vi "Insert data.vi"(8 "error in":errorcluster, 9 "Seleccion":T2, 10 "variant":variant, 11 "url":string) -> (0 "error out":errorcluster)   [LabVIEW 2018]
uses:
  Seleccion.ctl
  Valores Zapato.ctl
  Valores venta almacen.ctl
  Modelo color.ctl
  <vilib>/httpClient/POSTBuffer.vi
  <vilib>/httpClient/LabVIEWHTTPClient.lvlib
panel:
  out "JSON string":string
  out "data":T1[](array[typedef])
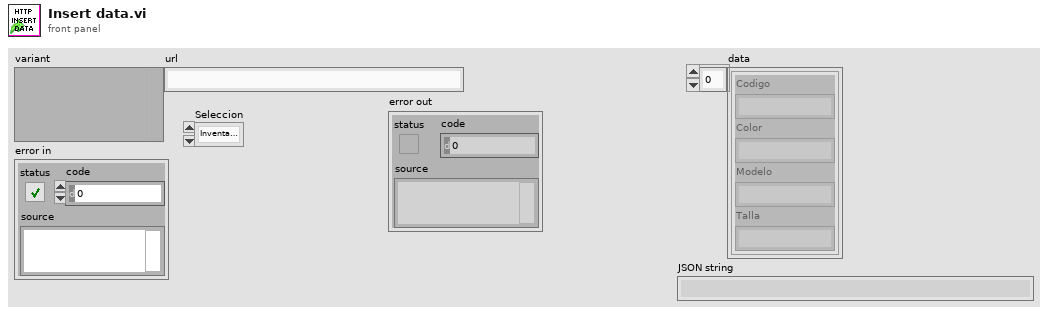
[diagram p1: front panel]
types:
  T1 = typedef "Valores Zapato.ctl" = cluster{"Codigo":string, "Color":string, "Modelo":string, "Talla":string}
  T2 = typedef "Seleccion.ctl" = enum16{"Inventario/ventas", "Zapatos", "Modelo/color"}
  T3 = typedef "Valores venta almacen.ctl" = cluster{"Cantidad":dbl, "Codigo":string, "Color":string, "Locacion/fecha":string, "Modelo":string, "Talla":string}
  T4 = typedef "Modelo color.ctl" = cluster{"Modelo/color":string}
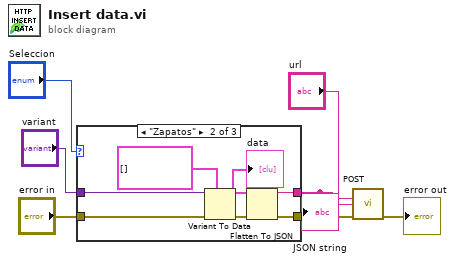
[diagram p0: block diagram]
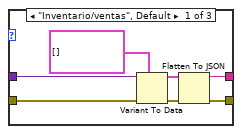
[diagram p2: hidden frame]
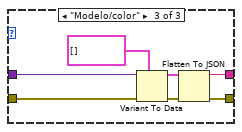
[diagram p3: hidden frame]
diagram:
  n1 = case shown="\"Zapatos\"" "Seleccion" {
    tunnel: [w9 w21 w28] -> w7
    tunnel: [w10 w20 w27] -> w6
    tunnel: "variant" -> [w12 w17 w24]
    tunnel: "error in" -> [w11 w16 w23]
    frame "Inventario/ventas", Default {
      n2 = Variant To Data(error in=w11, type=T3[] [], Variant=w12) -> (data=w13:T3[], error out=w14:errorcluster)
      n3 = Flatten To JSON(anything=w13, error in (no error)=w14) -> (JSON string=w10:string, 11:w9:errorcluster)  [unwired: 1 in]
    }
    frame "Zapatos" {
      n4 = Variant To Data(error in=w16, type=T1[] [], Variant=w17) -> (data=w18:T1[], error out=w19:errorcluster)
      "data" <- w18
      n5 = Flatten To JSON(anything=w18, error in (no error)=w19) -> (JSON string=w20:string, 11:w21:errorcluster)  [unwired: 1 in]
    }
    frame "Modelo/color" {
      n6 = Variant To Data(error in=w23, type=T4[] [], Variant=w24) -> (data=w25:T4[], error out=w26:errorcluster)
      n7 = Flatten To JSON(anything=w25, error in (no error)=w26) -> (JSON string=w27:string, 11:w28:errorcluster)  [unwired: 1 in]
    }
  }
  "JSON string" <- w6
  n8 = call-poly <vilib>:"POST.vi"("url"="url", "buffer"=w6, "error in (no error)"=w7) -> ("error out"=→"error out":errorcluster)  [unwired: 9 in, 3 out]
